vi "Go to Idle.vi"(8 "error in (no error)":errorcluster, 11 "Process State in":refnum<class "Process State.lvclass">) -> (0 "error out":errorcluster, 3 "Process State out":refnum<class "State Actor.lvclass">)   [LabVIEW 2014, in "States.lvlib" / "Process State.lvclass"]
doc: "This method defines the transition from any process state to the Idle state."
uses:
  Process State.lvclass
  <vilib>/NI/Actors/State Actor/State Actor/State Actor.lvclass
  Idle/Idle.lvclass
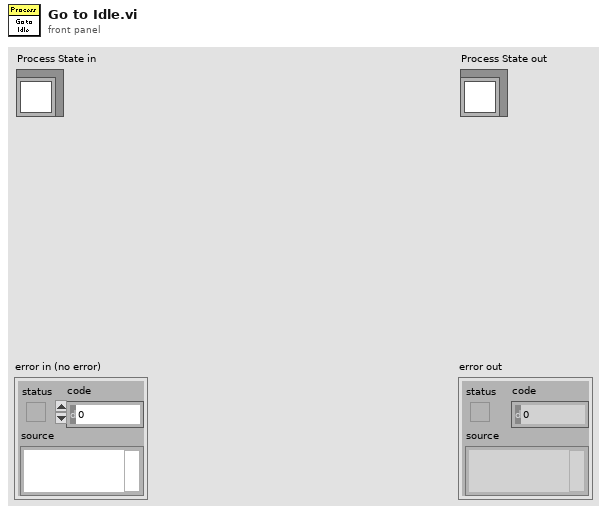
[diagram p1: front panel]
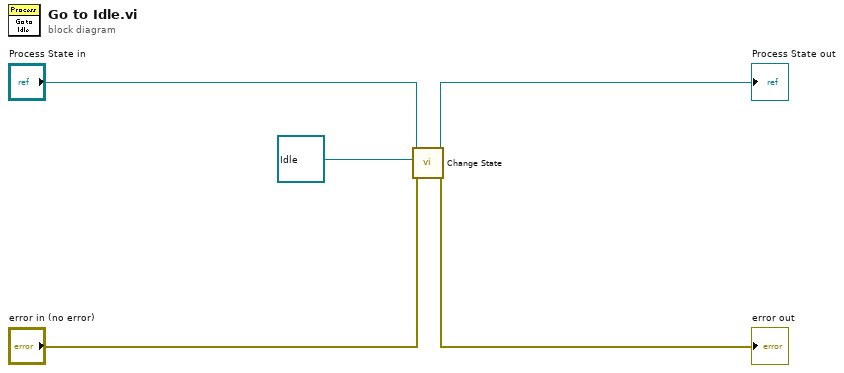
[diagram p0: block diagram]
diagram:
  n1 = call <vilib>:"Change State.vi"("error in (no error)"="error in (no error)", "New State in"=refnum<class "Idle.lvclass"> refnum ("Process States.lvlib:Ilde.lvclass"), "State in"="Process State in") -> ("error out"=→"error out":errorcluster, "State out"=→"Process State out":refnum<class "State Actor.lvclass">)  [unwired: 7 in]
